vi "Parse Persisted Bool Array.vi"(11 "file string value":string) -> (2 "valid":bool, 3 "Array of Booleans":bool[](array[boolean]))   [LabVIEW 2017]
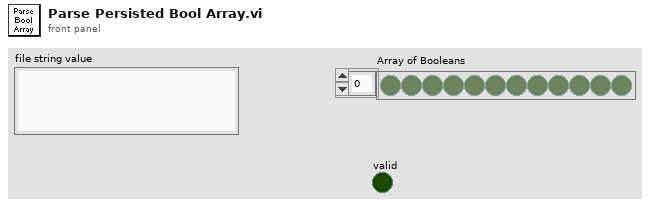
[diagram p1: front panel]
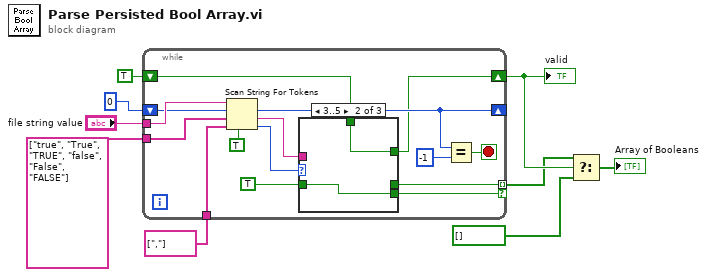
[diagram p0: block diagram]
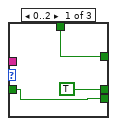
[diagram p2: hidden frame]
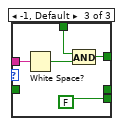
[diagram p3: hidden frame]
diagram:
  n1 = while {
    tunnel: "file string value" -> [w24]
    shift-right: [w19] -> _
    shift-left: 0 -> [w23]
    tunnel: string[] [","] ("delimiters (\\s,\\t,\\r,\\n)") -> [w22]
    tunnel: string[] ["true", "True", "TRUE", "false", "False", "FALSE"] ("delimiters (\\s,\\t,\\r,\\n)") -> [w21]
    tunnel: [w14] -> w1 mode=indexing if=w13
    shift-right: [w10] -> w4
    shift-left: TRUE ("use cached delim/oper data? (F)") -> [w11]
    stop <- w18 stop-if-true
    n2 = Scan String For Tokens(4:TRUE ("use cached delim/oper data? (F)"), 6:w22, 7:w21, 8:w23, 9:w24) -> (0:w16:i32, 1:w12:string, 2:w19:i32)  [unwired: 1 in, 1 out]
    n3 = case shown="3..5" w16 {
      tunnel: TRUE -> [w26 w29 _]
      tunnel: [TRUE _ _] -> w14
      tunnel: [w26 w29 FALSE] -> w13
      tunnel: w12 -> [_ _ w33]
      tunnel: [w25 w28 w30] -> w10
      tunnel: w11 -> [w25 w28 w31]
      frame 0..2 {
      }
      frame 3..5 {
      }
      frame -1, Default {
        n4 = White Space?(1:w33) -> (0:w32:bool)
        n5 = And(x=w31, y=w32) -> (x .and. y?=w30:bool)
      }
    }
    n6 = Equal?(x=w19, y=-1) -> (x = y?=w18:bool)
  }
  "valid" <- w4
  n7 = Select(t=w1, s=w4, f=bool[] []) -> (s? t:f=→"Array of Booleans":bool[])
